vi "Get Channels from Line.vi"(11 "Line":T1) -> (3 "Array":refnum<class "TBM channel.lvclass">[](array[class]))   [LabVIEW 2017, in "CentralErrorHandler configuration.lvclass"]
uses:
  CentralErrorHandler configuration.lvclass
  <vilib>/NI/Tag Bus Module Framework/channel/TBM channel.lvclass
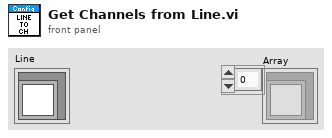
[diagram p1: front panel]
types:
  T1 = cluster{"channel":refnum<class "TBM channel.lvclass">}
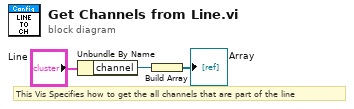
[diagram p0: block diagram]
diagram:
  # "This Vis Specifies how to get the all channels that are part of the line"
  n1 = Unbundle By Name("Line") -> ("channel"=w3:refnum<class "TBM channel.lvclass">)
  n2 = Build Array(w3) -> (→"Array":refnum<class "TBM channel.lvclass">[])
